vi "Write Tipo Motor.vi"(8 "error in (no error)":errorcluster, 10 "Tipo Motor":enum16{"Eléctrico", "Gasolina"}(ring), 11 "Vehiculo de Motor in":refnum<class "Vehiculo de Motor.lvclass">) -> (0 "error out":errorcluster, 3 "Vehiculo de Motor out":refnum<class "Vehiculo de Motor.lvclass">)   [LabVIEW 2020, in "Vehiculo de Motor.lvclass"]
uses:
  Vehiculo de Motor.lvclass
  Vehiculo de Motor.lvclass/Vehiculo de Motor.ctl
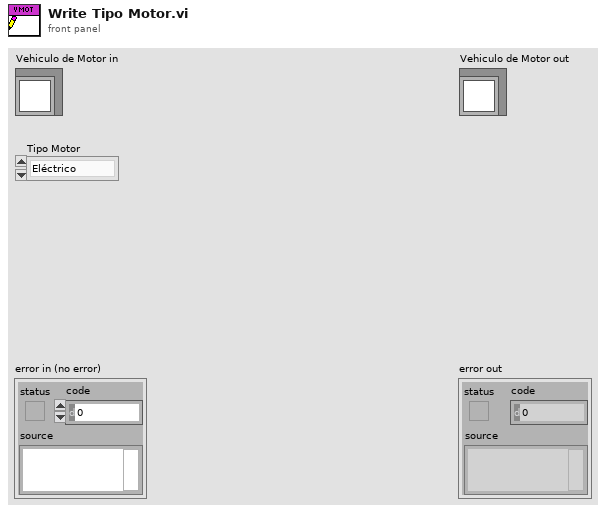
[diagram p1: front panel]
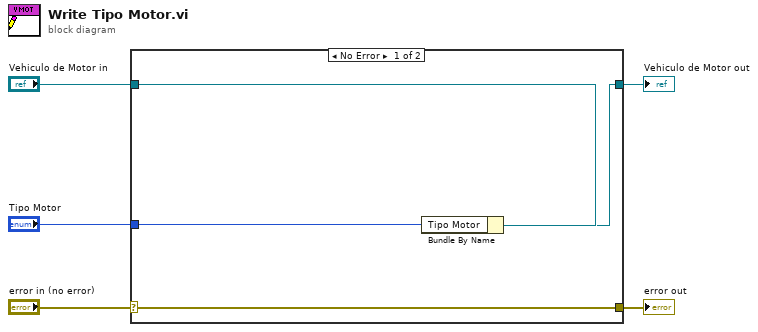
[diagram p0: block diagram]
diagram:
  n1 = case shown="No Error" "error in (no error)" {
    selector: "error in (no error)" -> [w9 w10]
    tunnel: [w9 w10] -> w4
    tunnel: [w7 w11] -> w2
    tunnel: "Vehiculo de Motor in" -> [w8 w11]
    tunnel: "Tipo Motor" -> [w6 _]
    frame No Error {
      n2 = Bundle By Name(cluster=w8, "Tipo Motor"=w6) -> (w7:refnum<class "Vehiculo de Motor.lvclass">)
    }
    frame Error {
    }
  }
  "error out" <- w4
  "Vehiculo de Motor out" <- w2
